vi "irrad calc u_prime v_prime.vi"(8 "error in (no error)":errorcluster, 10 "IRRAD Input Parameters":T2, 11 "Color Parameters in":T1) -> (0 "error out":errorcluster, 2 "IRRAD Input Parameters out":T2, 3 "Color Parameters out":T1)   [LabVIEW 2013, in "AvaSpec.lvlib" / "AVSirrad_support.lvlib"]
uses:
  AVSirrad_support.lvlib
  IRRAD input parameters.ctl
  Acquisition/AvaSpec Color Parameters.ctl
  <vilib>/express/express arith-compare/Formula/XNode/ExpressFormulaBlockNode.xnode
  AvaSpec.lvlib
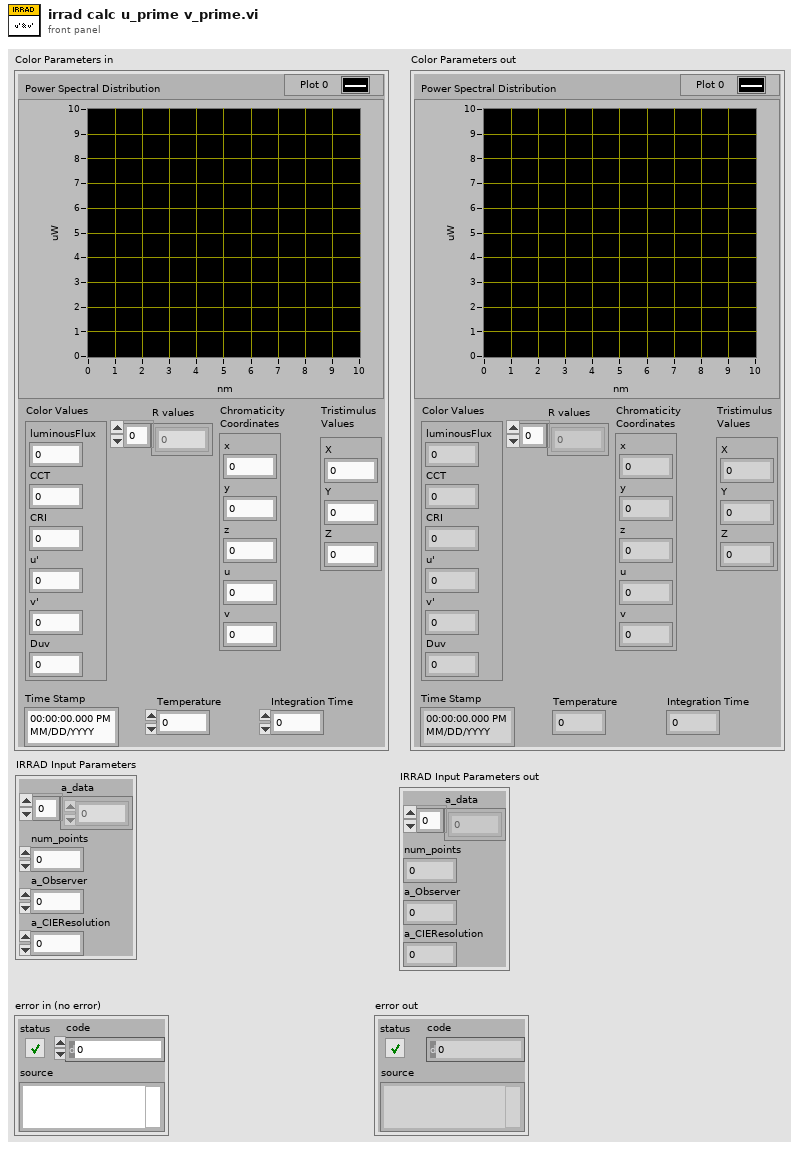
[diagram p1: front panel]
types:
  T1 = typedef "AvaSpec.lvlib/AvaSpec Color Parameters.ctl" = cluster{"Power Spectral Distribution":cluster{"X":dbl, "Y":dbl}[], "Color Values":cluster{"luminousFlux":dbl, "CCT":dbl, "CRI":dbl, "u'":dbl, "v'":dbl, "Duv":dbl}, "R values":dbl[], "Chromaticity \nCoordinates":cluster{"x":dbl, "y":dbl, "z":dbl, "u":dbl, "v":dbl}, "Tristimulus \nValues":cluster{"X":dbl, "Y":dbl, "Z":dbl}, "Time Stamp":timestamp, "Temperature":dbl, "Integration Time":dbl}
  T2 = typedef "IRRAD input parameters.ctl" = cluster{"a_data":dbl[], "num_points":i32, "a_Observer":u8, "a_CIEResolution":u8}
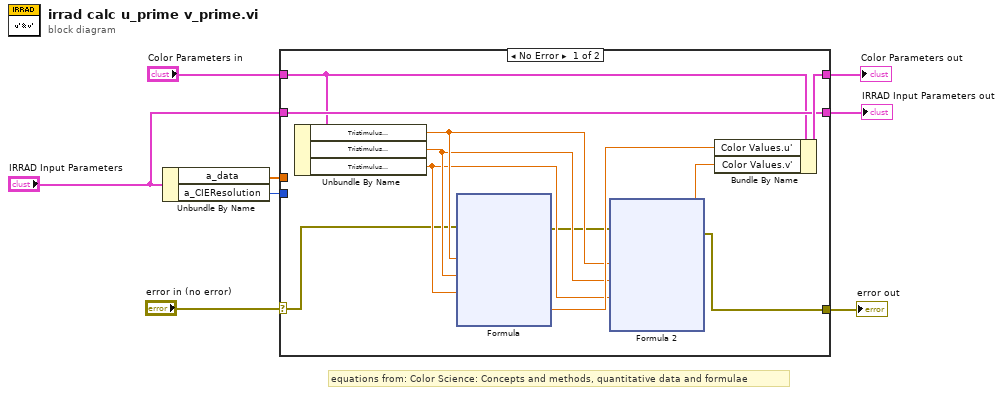
[diagram p0: block diagram]
diagram:
  # "equations from: Color Science: Concepts and methods, quantitative data and formulae"
  n1 = Unbundle By Name("IRRAD Input Parameters") -> ("a_data"=w5:dbl[], "a_CIEResolution"=w8:u8)
  n2 = case shown="No Error" "error in (no error)" {
    selector: "error in (no error)" -> [w11 w46]
    tunnel: [w9 w46] -> w2
    tunnel: w8 -> [_ _]
    tunnel: "Color Parameters in" -> [w17 w45]
    tunnel: [w19 w45] -> w4
    tunnel: w5 -> [_ _]
    tunnel: "IRRAD Input Parameters" -> [w18 w44]
    tunnel: [w18 w44] -> w7
    frame No Error {
      n3 = Unbundle By Name(w17) -> ("Tristimulus \nValues.X"=w15:dbl, "Tristimulus \nValues.Y"=w14:dbl, "Tristimulus \nValues.Z"=w13:dbl)
      n4 = xnode ("Formula")("X"=w15, "Y"=w14, "Z"=w13, "error in (no error)"=w11) -> ("Result"=w16:dbl, "error out"=w10:errorcluster)
      n5 = xnode ("Formula 2")("X"=w15, "Y"=w14, "Z"=w13, "error in (no error)"=w10) -> ("Result"=w12:dbl, "error out"=w9:errorcluster)
      n6 = Bundle By Name(cluster=w17, "Color Values.u'"=w16, "Color Values.v'"=w12) -> (w19:T1)
    }
    frame Error {
    }
  }
  "error out" <- w2
  "Color Parameters out" <- w4
  "IRRAD Input Parameters out" <- w7
